vi "GDSFile_SaveViCopy.vi"(6 "BackupFolder":path, 8 "error in":errorcluster, 9 "OverWirite(False)":bool, 10 "NewCopyPath":path, 11 "VIRef":refnum<vi>) -> (0 "error out":errorcluster, 1 "OverWritten":bool, 2 "BackupFileName":path)   [LabVIEW 2020, in "ClassWriterNative.lvclass"]
uses:
  <resource>/Framework/Providers/Open_GDS/ClassProviders/Provider_LvNativeClass/ClassWriterNative_class/ClassWriterNative.lvclass
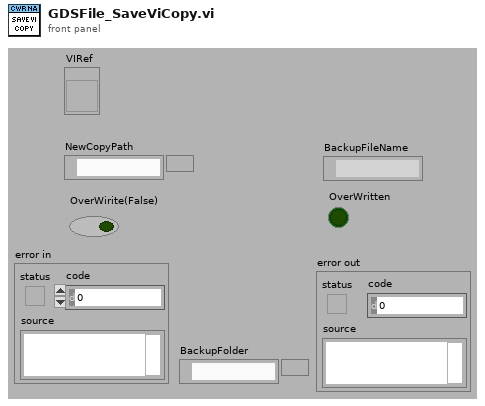
[diagram p1: front panel]
types:
  T1 = cluster{"App":refnum<vi>, "BackupFileName":path, "Overwrite":bool}
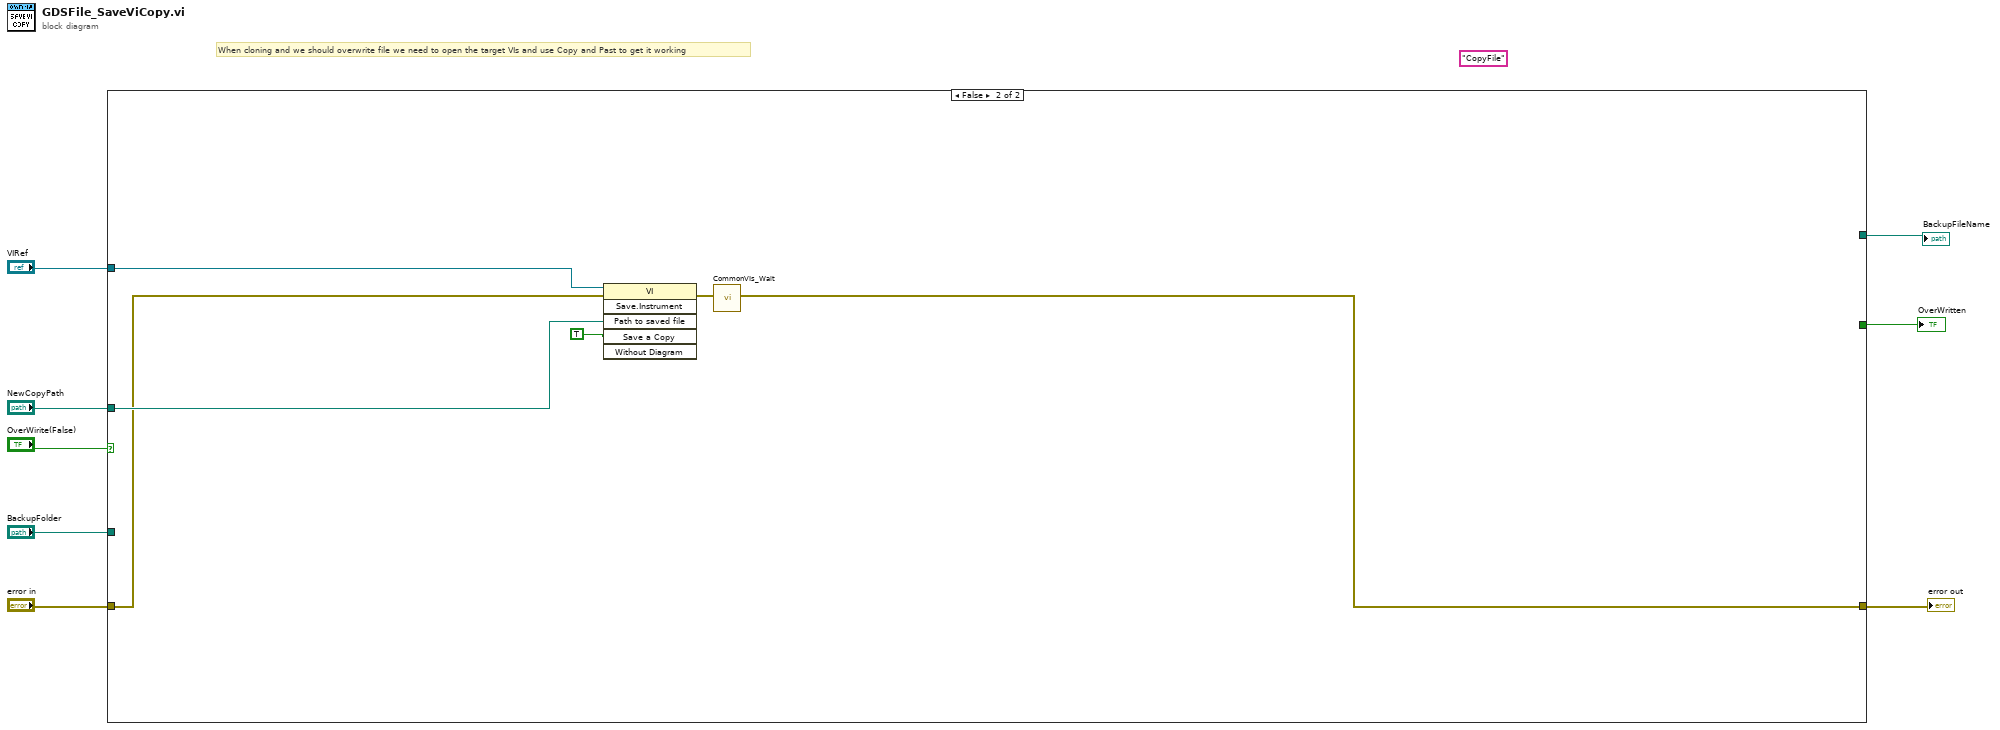
[diagram p0: block diagram]
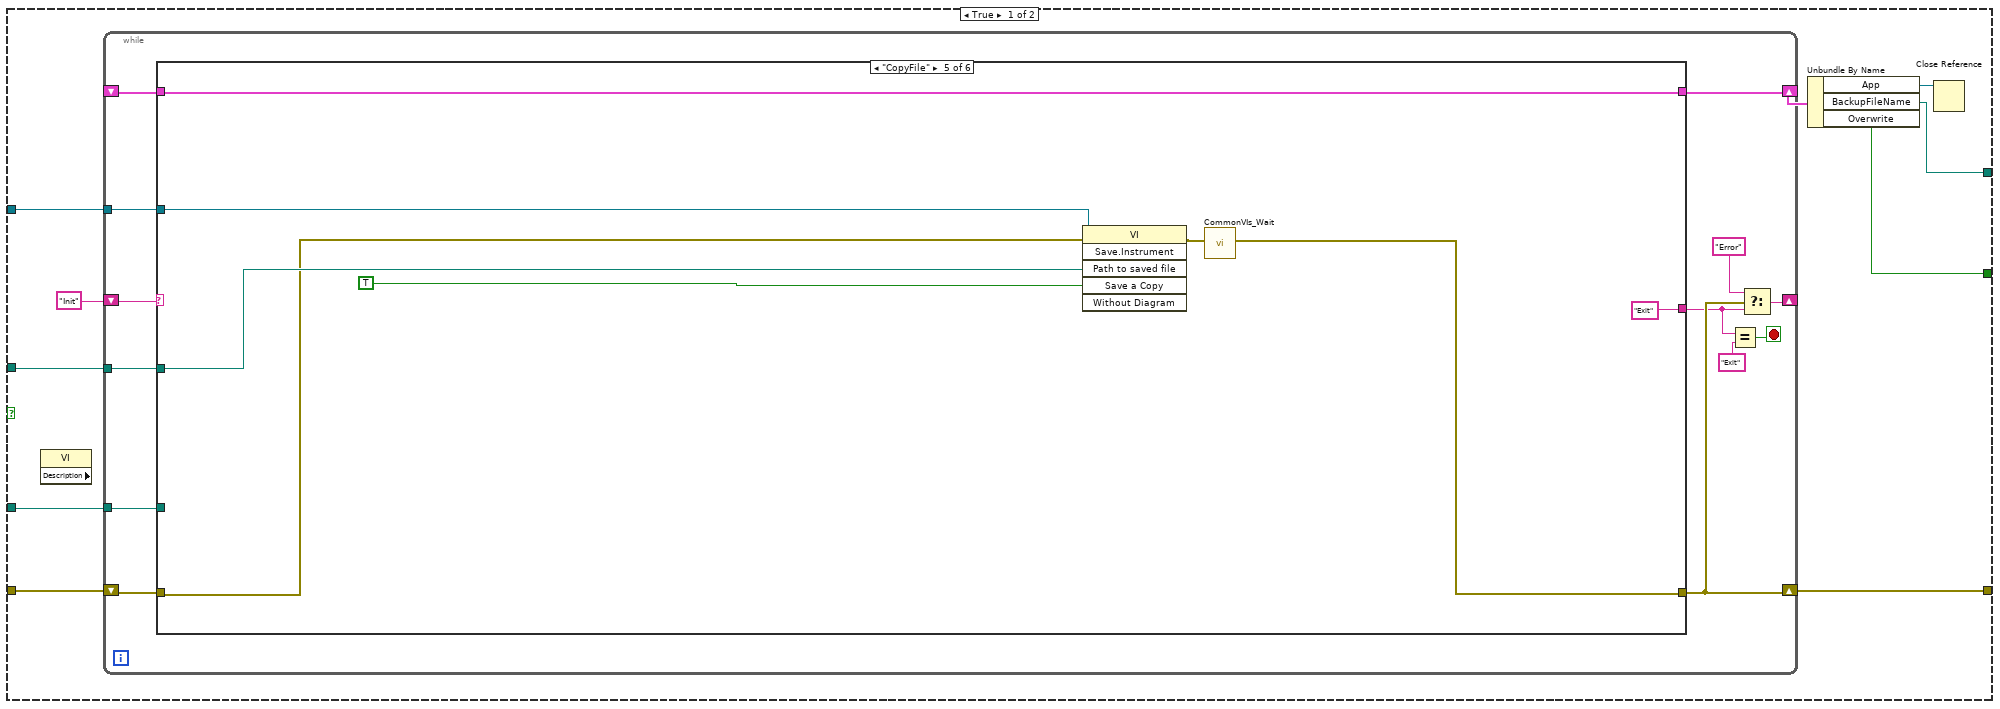
[diagram p2: hidden frame]
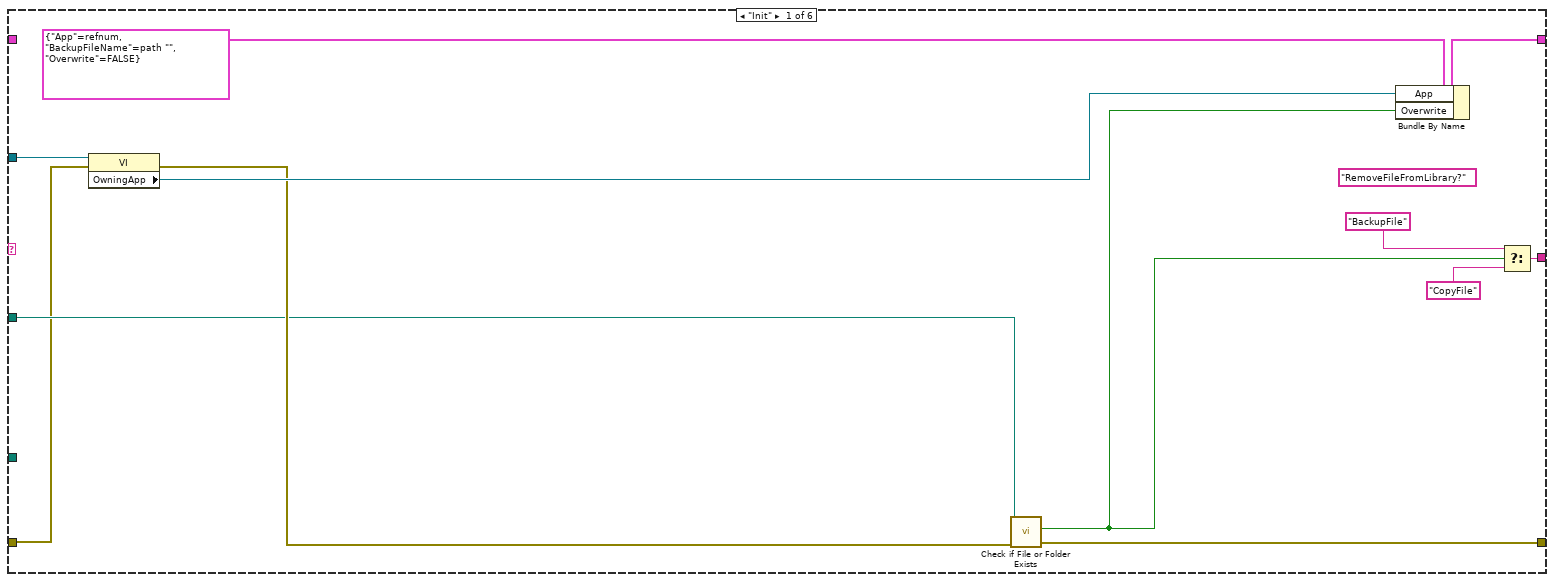
[diagram p3: hidden frame]
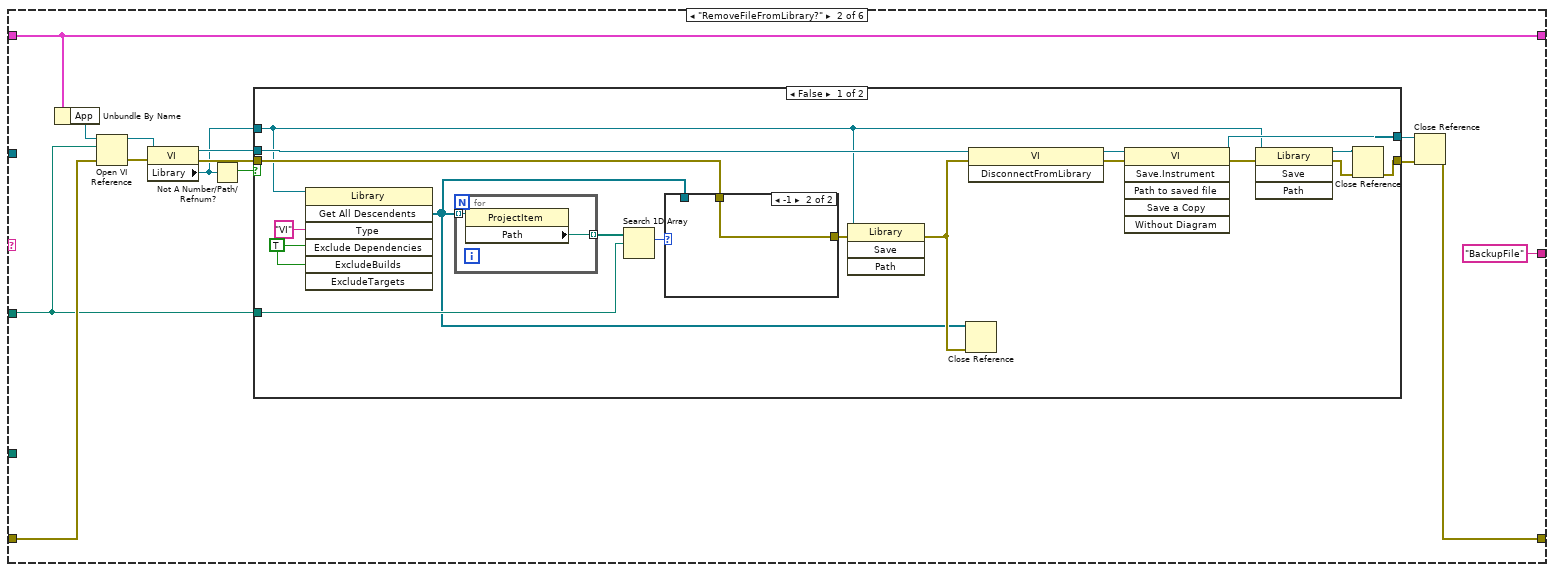
[diagram p4: hidden frame]
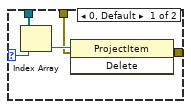
[diagram p5: hidden frame]
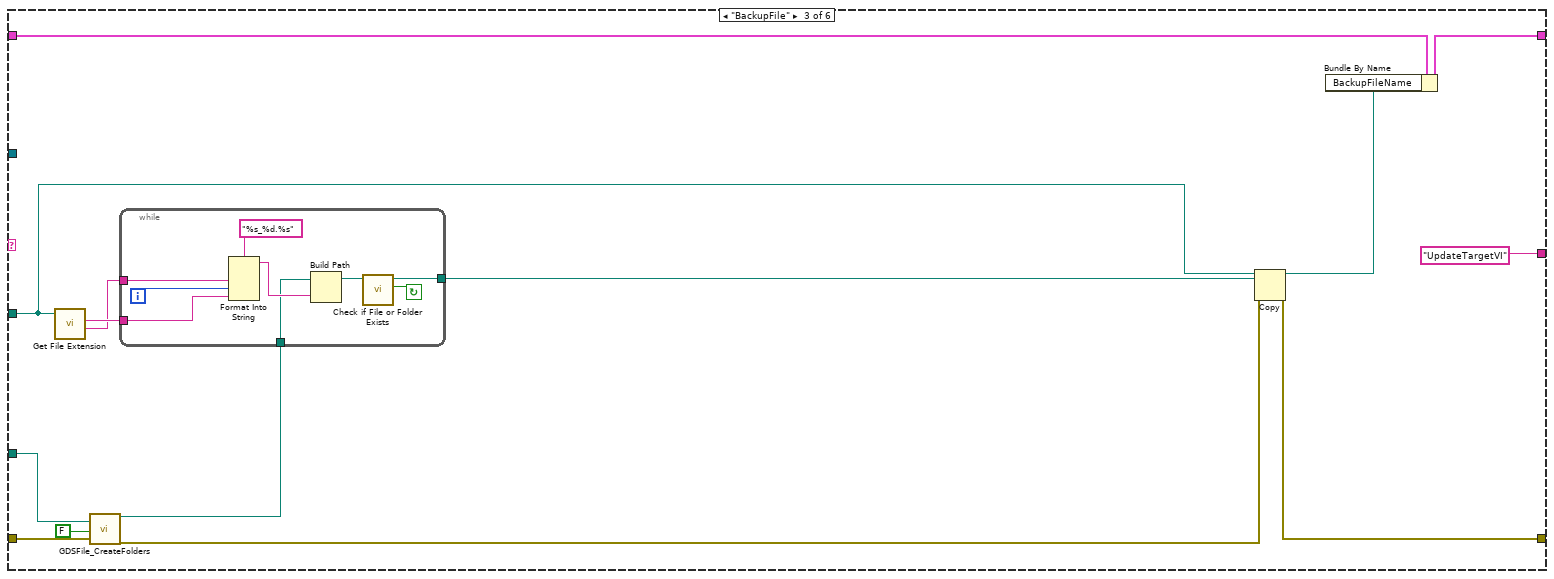
[diagram p7: hidden frame]
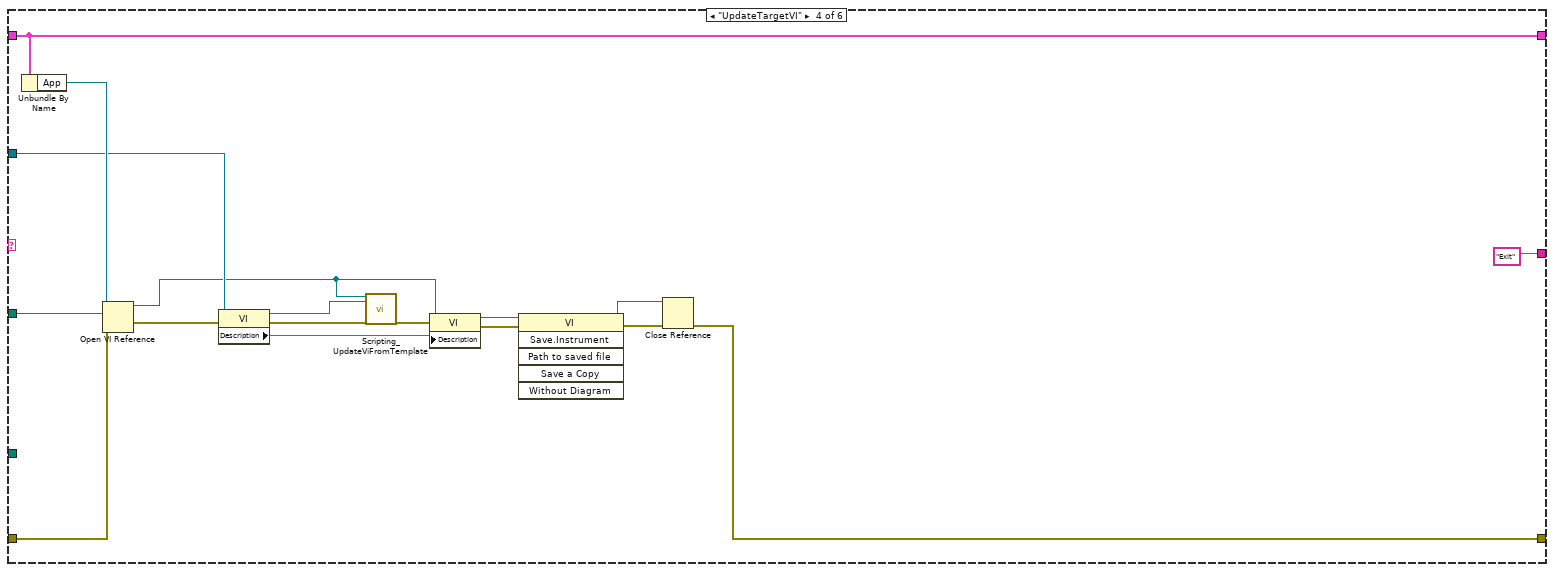
[diagram p8: hidden frame]
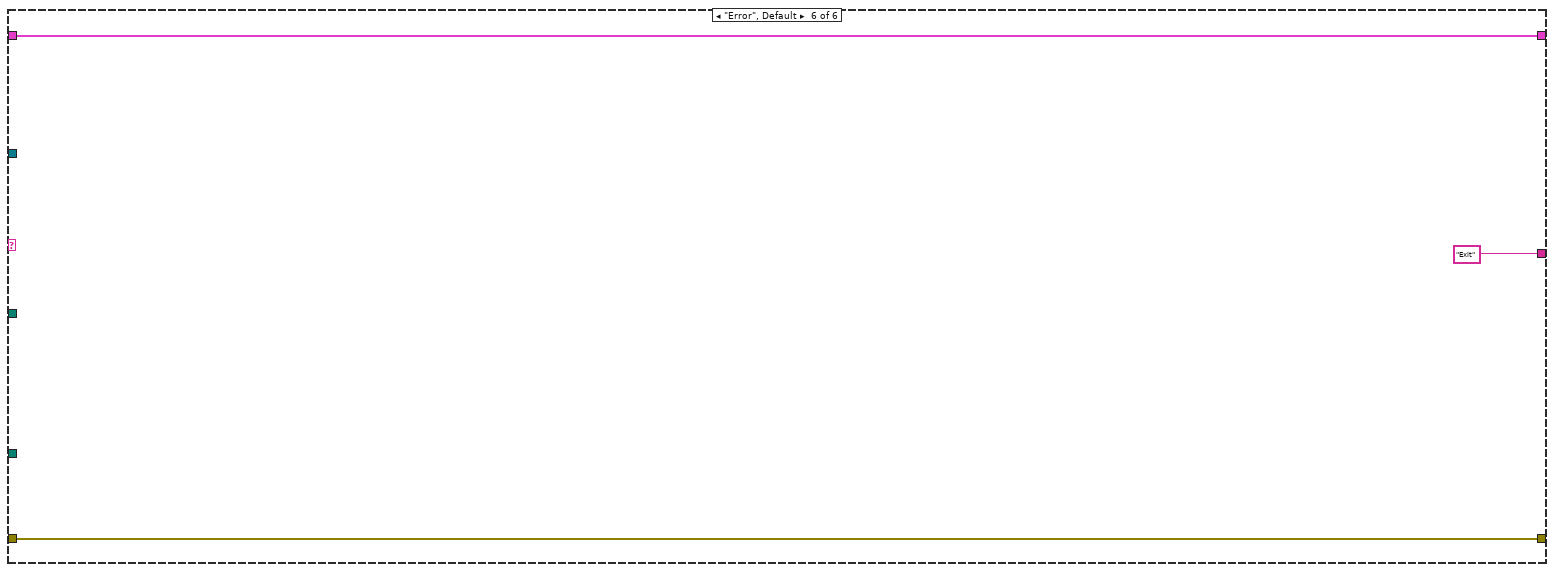
[diagram p9: hidden frame]
diagram:
  (unwired) "CopyFile"
  # "When cloning and we should overwrite file we need to open the target VIs and use Copy and Past to get it working"
  n1 = case shown="False" "OverWirite(False)" {
    tunnel: "NewCopyPath" -> [w14 w142]
    tunnel: [w15 w137] -> w7
    tunnel: "error in" -> [w18 w141]
    tunnel: "VIRef" -> [w16 w139]
    tunnel: "BackupFolder" -> [w11 _]
    tunnel: [w10 _] -> w2
    tunnel: [w9 _] -> w1
    frame True {
      n2 = property class="VI" props=["Description"]() -> ()  [unwired: 2 in, 3 out]
      n3 = while {
        shift-right: [w29] -> w15
        shift-left: w18 -> [w30]
        shift-right: [w25] -> _
        shift-left: "Init" -> [w31]
        shift-right: [w22] -> w12
        shift-left: _ -> [w20]
        tunnel: w16 -> [w23]
        tunnel: w14 -> [w21]
        tunnel: w11 -> [w19]
        stop <- w28 stop-if-true
        n4 = case shown="\"CopyFile\"" w31 {
          tunnel: [w35 w46 w90 w111 w126 w136] -> w29
          tunnel: w30 -> [w34 w55 w97 w123 w130 w136]
          tunnel: [w37 "BackupFile" ("t") "UpdateTargetVI" "Exit" "Exit" ("t") "Exit"] -> w24
          tunnel: w23 -> [w43 _ _ w121 w132 _]
          tunnel: [w41 w56 w88 w113 w128 w134] -> w22
          tunnel: w21 -> [w38 w44 w92 w125 w131 _]
          tunnel: w20 -> [_ w56 w89 w113 w128 w134]
          tunnel: w19 -> [_ _ w95 _ _ _]
          frame "Init" {
            (unwired) "RemoveFileFromLibrary?"
            n5 = property class="VI"(reference=w43, error in=w34) -> (error out=w39:errorcluster, "OwningApp"=w40:refnum<vi>)  [unwired: 1 out]
            n6 = call <vilib>:"Check if File or Folder Exists.vi"("error in (no error)"=w39, "path"=w38) -> ("error out"=w35:errorcluster, "file or folder exists?"=w32:bool)  [unwired: 7 in, 1 out]
            n7 = Bundle By Name(cluster=T1 {"App"=refnum, "BackupFileName"=path "", "Overwrite"=FALSE}, "App"=w40, "Overwrite"=w32) -> (w41:T1)
            n8 = Select(t="BackupFile", s=w32, f="CopyFile") -> (s? t:f=w37:string)
          }
          frame "RemoveFileFromLibrary?" {
            n9 = Unbundle By Name(w56) -> ("App"=w54:refnum<vi>)
            n10 = Open VI Reference(application reference (local)=w54, vi path=w44, error in (no error)=w55) -> (vi reference=w52:refnum<vi>, error out=w53:errorcluster)  [unwired: 3 in]
            n11 = property class="VI"(reference=w52, error in=w53) -> (reference out=w49:refnum<vi>, error out=w50:errorcluster, "Library"=w45:refnum<vi>)
            n12 = Not A Number/Path/Refnum?(number/path/refnum=w45) -> (NaN/Path/Refnum?=w51:bool)
            n13 = case shown="False" w51 {
              tunnel: w50 -> [w63 w85]
              tunnel: w49 -> [w73 w84]
              tunnel: [w68 w85] -> w48
              tunnel: [w71 w84] -> w47
              tunnel: w45 -> [w61 _]
              tunnel: w44 -> [w64 _]
              frame False {
                w67 = TRUE ("ExcludeDependencies")
                n14 = invoke class="Library" method="Get All Descendents"(reference=w61, "Type"="VI", "Exclude Dependencies"=w67, "ExcludeBuilds"=w67) -> ("All Descendents"=w59:refnum<vi>[])  [unwired: 3 in, 6 out]
                n15 = for {
                  tunnel: w59 -> [w83] mode=indexing
                  tunnel: [w82] -> w65 mode=indexing
                  n16 = property class="ProjectItem"(reference=w83) -> ("Path"=w82:path)  [unwired: 1 in, 2 out]
                }
                n17 = Search 1D Array(1D array=w65, element=w64) -> (index of element=w58:i32)  [unwired: 1 in]
                n18 = case shown="-1" w58 {
                  selector: w58 -> [w76 _]
                  tunnel: w63 -> [w79 w81]
                  tunnel: [w78 w81] -> w62
                  tunnel: w59 -> [w77 _]
                  frame 0, Default {
                    n19 = Index Array(array=w77, index=w76) -> (element=w80:refnum<vi>)
                    n20 = invoke class="ProjectItem" method="Delete"(reference=w80, error in=w79) -> (error out=w78:errorcluster)  [unwired: 1 in, 2 out]
                  }
                  frame -1 {
                  }
                }
                n21 = invoke class="Library" method="Save"(reference=w61, error in=w62) -> (error out=w60:errorcluster)  [unwired: 2 in, 3 out]
                n22 = Close Reference(reference=w59, error in (no error)=w60) -> ()  [unwired: 1 out]
                n23 = invoke class="VI" method="DisconnectFromLibrary"(reference=w73, error in=w60) -> (reference out=w72:refnum<vi>, error out=w75:errorcluster)  [unwired: 1 in, 1 out]
                n24 = invoke class="VI" method="Save.Instrument"(reference=w72, error in=w75) -> (reference out=w71:refnum<vi>, error out=w74:errorcluster)  [unwired: 4 in, 4 out]
                n25 = invoke class="Library" method="Save"(reference=w61, error in=w74) -> (reference out=w70:refnum<vi>, error out=w69:errorcluster)  [unwired: 2 in, 2 out]
                n26 = Close Reference(reference=w70, error in (no error)=w69) -> (error out=w68:errorcluster)
              }
              frame True {
              }
            }
            n27 = Close Reference(reference=w47, error in (no error)=w48) -> (error out=w46:errorcluster)
          }
          frame "BackupFile" {
            n28 = call <vilib>:"Get File Extension.vi"("file"=w92) -> ("filename without extension"=w98:string, "lowercase file extension"=w99:string)  [unwired: 6 in, 3 out]
            n29 = call <resource>:"GDSFile_CreateFolders.vi"("Path"=w95, "Promt if folder\ndoes not exists?"=FALSE ("Promt if folder\ndoes not exists?"), "error in (no error)"=w97) -> ("PathOut"=w94:path, "error out"=w93:errorcluster)  [unwired: 12 in, 3 out]
            n30 = while {
              tunnel: w94 -> [w106]
              tunnel: w98 -> [w105]
              tunnel: w99 -> [w103]
              tunnel: [w100] -> w91
              i -> [w104]
              stop <- w101 continue-if-true
              n31 = Format Into String(format string="%s_%d.%s", w105, w104, w103) -> (resulting string=w107:string)  [unwired: 2 in, 1 out]
              n32 = Build Path(base path=w106, name or relative path=w107) -> (appended path=w102:path)
              n33 = call <vilib>:"Check if File or Folder Exists.vi"("path"=w102) -> ("file or folder exists?"=w101:bool, "dup path"=w100:path)  [unwired: 8 in, 1 out]
            }
            n34 = Copy(8:w93, 10:w91, 11:w92) -> (0:w90:errorcluster, 3:w87:path)  [unwired: 2 in, 1 out]
            n35 = Bundle By Name(cluster=w89, "BackupFileName"=w87) -> (w88:T1)
          }
          frame "UpdateTargetVI" {
            n36 = Unbundle By Name(w113) -> ("App"=w124:refnum<vi>)
            n37 = Open VI Reference(application reference (local)=w124, vi path=w125, error in (no error)=w123) -> (vi reference=w117:refnum<vi>, error out=w120:errorcluster)  [unwired: 3 in]
            n38 = property class="VI"(reference=w121, error in=w120) -> (reference out=w119:refnum<vi>, error out=w118:errorcluster, "Description"=w116:string)
            n39 = call <resource>:"Scripting_UpdateViFromTemplate.vi"("ViRef"=w117, "TemplateVI(Path or Ref)"=w119, "error in (no error)"=w118) -> ("error out"=w122:errorcluster)  [unwired: 15 in, 1 out]
            n40 = property class="VI"(reference=w117, error in=w122, "Description"=w116) -> (reference out=w115:refnum<vi>, error out=w114:errorcluster)
            n41 = invoke class="VI" method="Save.Instrument"(reference=w115, error in=w114) -> (reference out=w110:refnum<vi>, error out=w112:errorcluster)  [unwired: 4 in, 4 out]
            n42 = Close Reference(reference=w110, error in (no error)=w112) -> (error out=w111:errorcluster)
          }
          frame "CopyFile" {
            n43 = invoke class="VI" method="Save.Instrument"(reference=w132, error in=w130, "Path to saved file"=w131, "Save a Copy"=TRUE) -> (error out=w127:errorcluster)  [unwired: 2 in, 5 out]
            n44 = call <resource>:"CommonVIs_Wait.vi"("error in"=w127) -> ("error out"=w126:errorcluster)  [unwired: 9 in]
          }
          frame "Error", Default {
          }
        }
        n45 = Equal?(x=w24, y="Exit") -> (x = y?=w28:bool)
        n46 = Select(t="Error", s=w29, f=w24) -> (s? t:f=w25:string)
      }
      n47 = Unbundle By Name(w12) -> ("App"=w13:refnum<vi>, "BackupFileName"=w10:path, "Overwrite"=w9:bool)
      n48 = Close Reference(reference=w13) -> ()  [unwired: 1 in, 1 out]
    }
    frame False {
      n49 = invoke class="VI" method="Save.Instrument"(reference=w139, error in=w141, "Path to saved file"=w142, "Save a Copy"=TRUE) -> (error out=w138:errorcluster)  [unwired: 2 in, 5 out]
      n50 = call <resource>:"CommonVIs_Wait.vi"("error in"=w138) -> ("error out"=w137:errorcluster)  [unwired: 9 in]
    }
  }
  "error out" <- w7
  "BackupFileName" <- w2
  "OverWritten" <- w1
